vi "ThreeIncoming_TwoDataTypes.vi"() -> ()   [LabVIEW 2015]
uses:
  <vilib>/rvi/Emulation/niFpgaGetClockAttributes.vi
  <vilib>/rvi/Emulation/niFpgaSctlEmulationGetInTimedLoop.vi
  <vilib>/rvi/Emulation/niFpgaEmulationReportErrorSimple.vi
  <vilib>/rvi/Emulation/niFpgaCriticalErrorInLSC.vi
  <vilib>/rvi/interface/RandomDataEmulation/niFpgaRandomDataHandleErrors.vi
  <vilib>/rvi/DataTransferAndStorage/Container/XNode/niFpgaContainer.xnode
  <vilib>/rvi/interface/RandomDataEmulation/nirviRandomDataFpgaReadWriteTemplate.vi
panel:
  in  "FXP27.5":fxp<+/-,27,5>
  out "FXP27.5 out":fxp<+/-,27,5>
  in  "FXP20.5":fxp<+/-,20,5>
  out "FXP20.5 out":fxp<+/-,20,5>
  in  "FXP16.7":fxp<+/-,16,7>
  out "FXP16.7 out":fxp<+/-,16,7>
  out "FXP64.32 out":fxp<+/-,64,32>
  out "FXP32.8 out":fxp<+/-,32,8>
  out "FXP16.5 out":fxp<+/-,16,5>
  out "FXP24.5 out":fxp<+/-,24,5>
  in  "FXP64.32":fxp<+/-,64,32>
  in  "FXP32.8":fxp<+/-,32,8>
  in  "FXP16.5":fxp<+/-,16,5>
  in  "FXP24.5":fxp<+/-,24,5>
  out "Boolean 2":bool=TRUE
  out "Fast timeout":bool
  out "Med timeout":bool
  out "Slow timeout":bool
  in  "I16":i16
  in  "I8":i8
  in  "I64":i64
  in  "I32":i32
  in  "U16":u16
  in  "U8":u8
  in  "U64":u64
  in  "U32":u32
  in  "SGL":sgl
  in  "Boolean":bool
  out "I16 out":i16
  out "I8 out":i8
  out "I64 out":i64
  out "I32 out":i32
  out "U16 out":u16
  out "U8 out":u8
  out "U64 out":u64
  out "U32 out":u32
  out "SGL out":sgl
  out "Boolean out":bool
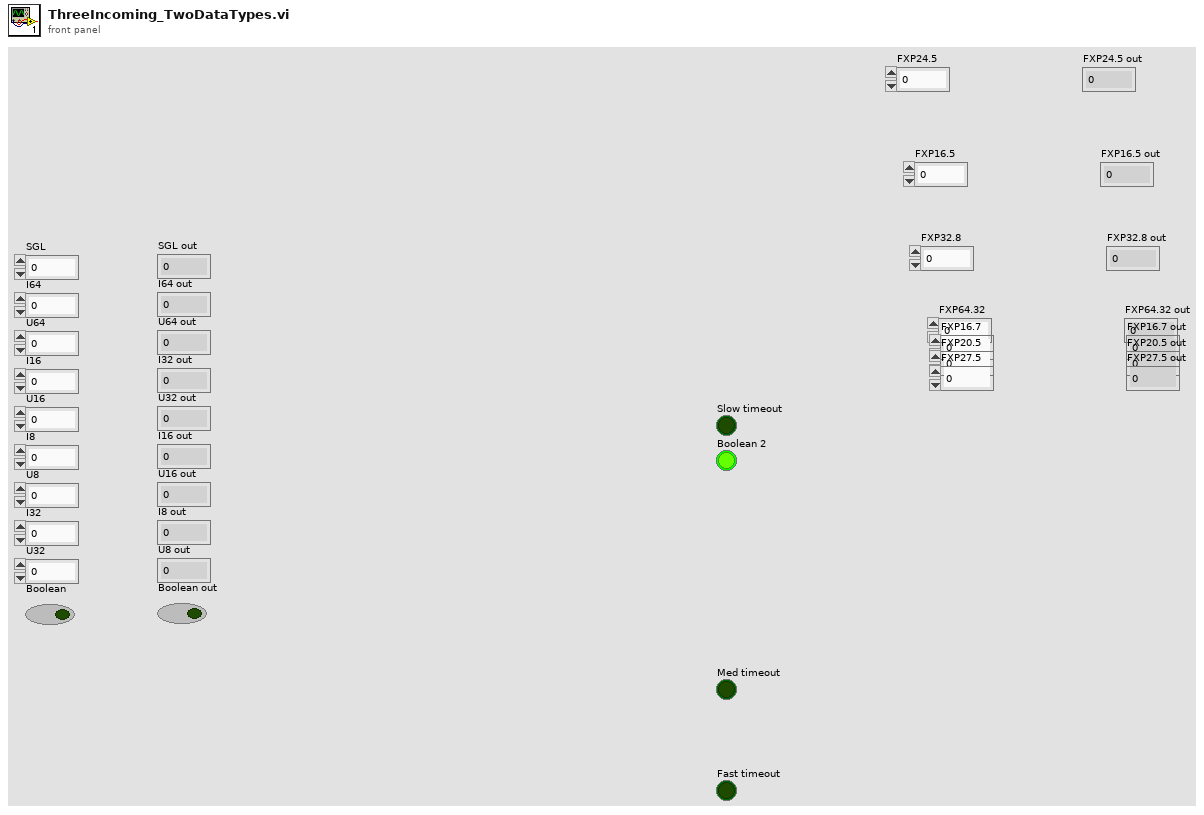
[diagram p1: front panel]
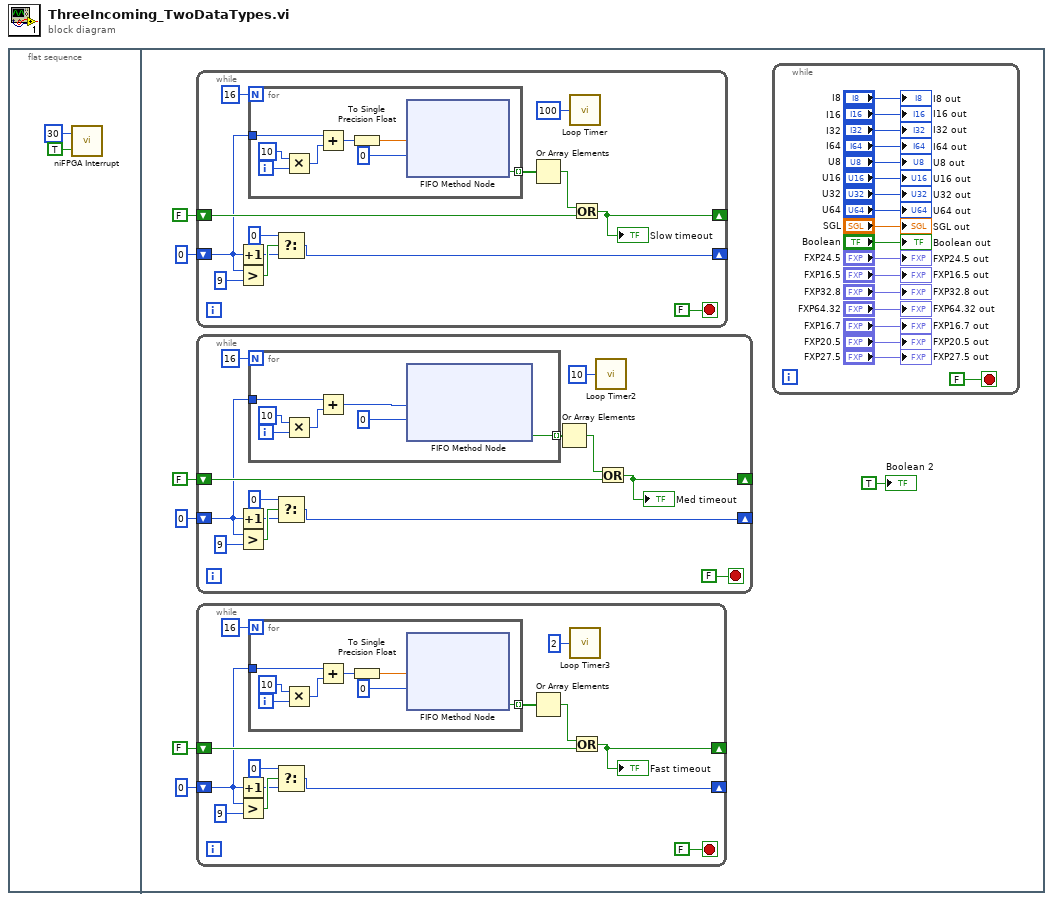
[diagram p0: block diagram]
diagram:
  n1 = flat-sequence {
    frame #0 {
      n2 = call <vilib>:"niFPGA Interrupt.vi"("Wait Until Cleared (F)"=TRUE, "IRQ Number (0)"=u8 30) -> ()  [unwired: 1 in]
    }
    frame #1 {
      n3 = while {
        shift-right: [w58] -> _
        shift-left: 0 ("t") -> [w51]
        shift-right: [w52] -> _
        shift-left: FALSE -> [w53]
        stop <- FALSE stop-if-true
        n4 = Increment(x=w51) -> (x+1=w56:i32)
        n5 = Greater?(x=w51, y=9) -> (0:w62:bool)
        n6 = for {
          N: 16 -> [_]
          tunnel: w51 -> [w71]
          tunnel: [w64] -> w55 mode=indexing
          i -> [w70]
          n7 = Multiply(x=10, y=w70) -> (x*y=w68:i32)
          n8 = Add(x=w71, y=w68) -> (x+y=w67:i32)
          n9 = To Single Precision Float(number=w67) -> (single precision float=w66:sgl)
          n10 = xnode ("FIFO Method Node")("Element"=w66, "Timeout"=0) -> ("Timed Out?"=w64:bool)  [unwired: 1 in, 1 out]
        }
        n11 = Select(t=0, s=w62, f=w56) -> (s? t:f=w58:i32)
        n12 = Or Array Elements(Boolean array=w55) -> (logical OR=w54:bool)
        n13 = call "Loop Timer"("Count(uSec)"=u32 100) -> ()  [unwired: 1 out]
        n14 = Or(x=w54, y=w53) -> (x .or. y?=w52:bool)
        "Slow timeout" <- w52
      }
      n15 = while {
        shift-right: [w38] -> _
        shift-left: 0 ("t") -> [w31]
        shift-right: [w32] -> _
        shift-left: FALSE -> [w33]
        stop <- FALSE stop-if-true
        n16 = Increment(x=w31) -> (x+1=w36:i32)
        n17 = Greater?(x=w31, y=9) -> (0:w42:bool)
        n18 = for {
          N: 16 -> [_]
          tunnel: w31 -> [w50]
          tunnel: [w45] -> w35 mode=indexing
          i -> [w49]
          n19 = Multiply(x=10, y=w49) -> (x*y=w47:i32)
          n20 = Add(x=w50, y=w47) -> (x+y=w44:i32)
          n21 = xnode ("FIFO Method Node")("Element"=w44, "Timeout"=0) -> ("Timed Out?"=w45:bool)  [unwired: 1 in, 1 out]
        }
        n22 = Select(t=0, s=w42, f=w36) -> (s? t:f=w38:i32)
        n23 = Or Array Elements(Boolean array=w35) -> (logical OR=w34:bool)
        n24 = call "Loop Timer2"("Count(uSec)"=u32 10) -> ()  [unwired: 1 out]
        n25 = Or(x=w34, y=w33) -> (x .or. y?=w32:bool)
        "Med timeout" <- w32
      }
      n26 = while {
        shift-right: [w17] -> _
        shift-left: 0 ("t") -> [w10]
        shift-right: [w11] -> _
        shift-left: FALSE -> [w12]
        stop <- FALSE stop-if-true
        n27 = Increment(x=w10) -> (x+1=w15:i32)
        n28 = Greater?(x=w10, y=9) -> (0:w21:bool)
        n29 = for {
          N: 16 -> [_]
          tunnel: w10 -> [w30]
          tunnel: [w23] -> w14 mode=indexing
          i -> [w29]
          n30 = Multiply(x=10, y=w29) -> (x*y=w27:i32)
          n31 = Add(x=w30, y=w27) -> (x+y=w26:i32)
          n32 = To Single Precision Float(number=w26) -> (single precision float=w25:sgl)
          n33 = xnode ("FIFO Method Node")("Element"=w25, "Timeout"=0) -> ("Timed Out?"=w23:bool)  [unwired: 1 in, 1 out]
        }
        n34 = Select(t=0, s=w21, f=w15) -> (s? t:f=w17:i32)
        n35 = Or Array Elements(Boolean array=w14) -> (logical OR=w13:bool)
        n36 = call "Loop Timer3"("Count(uSec)"=u32 2) -> ()  [unwired: 1 out]
        n37 = Or(x=w13, y=w12) -> (x .or. y?=w11:bool)
        "Fast timeout" <- w11
      }
      n38 = while {
        stop <- FALSE stop-if-true
        "I16 out" <- "I16"
        "I8 out" <- "I8"
        "I64 out" <- "I64"
        "I32 out" <- "I32"
        "U16 out" <- "U16"
        "U8 out" <- "U8"
        "U64 out" <- "U64"
        "U32 out" <- "U32"
        "SGL out" <- "SGL"
        "Boolean out" <- "Boolean"
        "FXP24.5 out" <- "FXP24.5"
        "FXP16.5 out" <- "FXP16.5"
        "FXP32.8 out" <- "FXP32.8"
        "FXP64.32 out" <- "FXP64.32"
        "FXP16.7 out" <- "FXP16.7"
        "FXP20.5 out" <- "FXP20.5"
        "FXP27.5 out" <- "FXP27.5"
      }
      "Boolean 2" <- TRUE
    }
  }
